vi "Available DMA FG.vi"(6 "Action":T4, 8 "error in (no error)":errorcluster, 10 "Available DMA":T1[](array[typedef]), 11 "Item Ref":T5 format="%.0x") -> (0 "error out":errorcluster, 2 "Available DMA":T1[](array[typedef]), 3 "Item Ref out":T5=18446744073709551615 format="%.0x")   [LabVIEW 2015, in "FPGA Addon Shared.lvlib"]
uses:
  FPGA Addon Shared.lvlib
  <vilib>/rvi/FIFO/Fifo_Types/Fifo_DMA_Config.ctl
  <vilib>/rvi/DataTransferAndStorage/Container/Common/niFpgaDataTypeControl.ctl
  <vilib>/rvi/ClientSDK/Core/ModuleGeneration/CommunicationInterfaceUtility/niFpgaDmaChannelImplementation.ctl
  <vilib>/NI Veristand/Custom Device API/Custom Device Item Ref.ctl
  FG Action.ctl
  <vilib>/NI Veristand/Custom Device API/Set Item Property (Variant).vi
  <vilib>/NI Veristand/Custom Device API/Get Item Property (Variant).vi
  Constants.vi
  <vilib>/NI VeriStand/Custom Device API/Custom Device API.lvlib
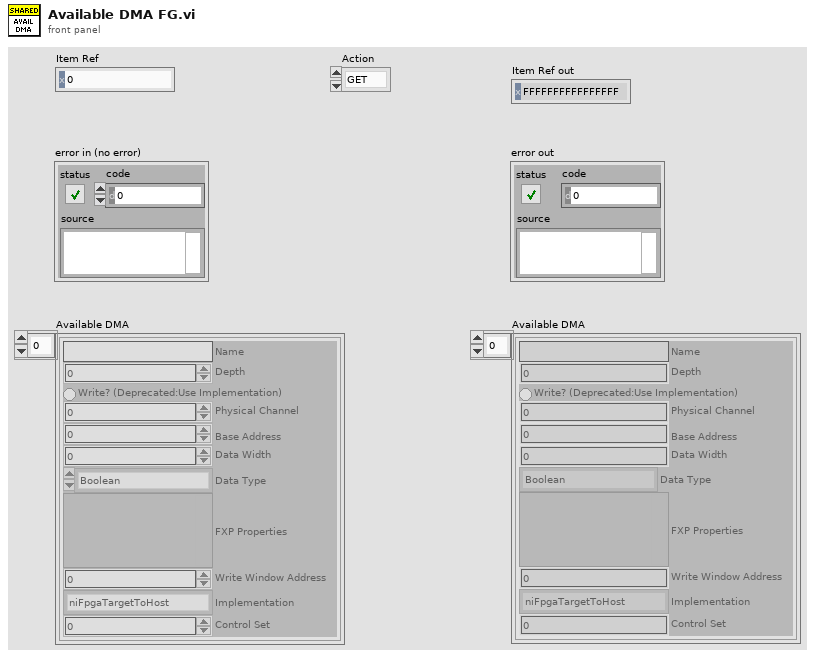
[diagram p1: front panel]
types:
  T1 = typedef "Fifo_DMA_Config.ctl" = cluster{"Name":string, "Depth":u32, "Write? (Deprecated:Use Implementation)":bool, "Physical Channel":u32, "Base Address":u32, "Data Width":u32, "Data Type":T2, "FXP Properties":variant, "Write Window Address":u32, "Implementation":T3, "Control Set":u32}
  T2 = typedef "niFpgaDataTypeControl.ctl" = enum32{"Boolean", "I8", "I16", "I32", "I64", "U8", "U16", "U32", "U64", "FXP", "CustomControl", "SGL"}
  T3 = typedef "niFpgaDmaChannelImplementation.ctl" = enum16{"niFpgaTargetToHost", "niFpgaHostToTarget", "niFpgaPeerToPeerWriter", "niFpgaPeerToPeerReader", "niCoreTargetToHost", "niCoreHostToTarget"}
  T4 = typedef "FPGA Addon Shared.lvlib/FG Action.ctl" = enum8{"GET", "SET"}
  T5 = typedef "Custom Device API.lvlib/Custom Device Item Ref.ctl" = u64
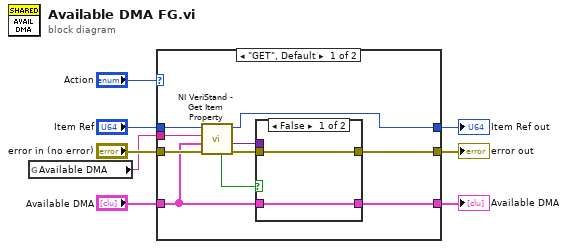
[diagram p0: block diagram]
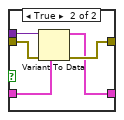
[diagram p2: hidden frame]
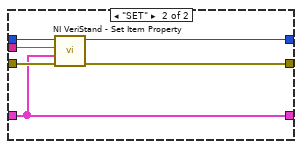
[diagram p3: hidden frame]
diagram:
  n1 = global read "Constants.vi" "Available DMA"() -> (w2:string)
  n2 = case shown="\"GET\", Default" "Action" {
    tunnel: "error in (no error)" -> [w18 w31]
    tunnel: "Item Ref" -> [w17 w30]
    tunnel: "Available DMA" -> [w15 w27]
    tunnel: [w13 w29] -> w8
    tunnel: [w10 w28] -> w4
    tunnel: [w11 w27] -> w1
    tunnel: w2 -> [w9 w26]
    frame "GET", Default {
      n3 = call-poly <vilib>:"NI VeriStand - Get Item Property.vi"("error in (no error)"=w18, "Default Value"=w15, "Property Name"=w9, "Item Ref in"=w17) -> ("error out"=w14:errorcluster, "Value"=w16:variant, "Item Ref out"=w10:T5, "Found?"=w12:bool)  [unwired: 4 in]
      n4 = case shown="False" w12 {
        tunnel: w16 -> [_ w25]
        tunnel: w15 -> [w19 w24]
        tunnel: w14 -> [w20 w23]
        tunnel: [w20 w22] -> w13
        tunnel: [w19 w21] -> w11
        frame False {
        }
        frame True {
          n5 = Variant To Data(error in=w23, type=w24, Variant=w25) -> (data=w21:T1[], error out=w22:errorcluster)
        }
      }
    }
    frame "SET" {
      n6 = call-poly <vilib>:"NI VeriStand - Set Item Property.vi"("error in (no error)"=w31, "Value"=w27, "Property Name"=w26, "Item Ref in"=w30) -> ("error out"=w29:errorcluster, "Item Ref out"=w28:T5)  [unwired: 5 in, 1 out]
    }
  }
  "error out" <- w8
  "Item Ref out" <- w4
  "Available DMA" <- w1
